vi "Rayleigh Inverse CDF.vi"(10 "b":dbl=3.0, 11 "cdf(x)":dbl=0.25) -> (0 "error":i32, 3 "x":dbl=2.275582849322796)   [LabVIEW 2010, in "NI_Gmath.lvlib"]
doc: "Computes the continuous inverse cumulative distribution function (CDF) of the various distributions. You must manually select the polymorphic instance to use."
uses:
  NI_Gmath.lvlib
  st_error_code.ctl
panel:
  # "Rayleigh Inverse CDF"
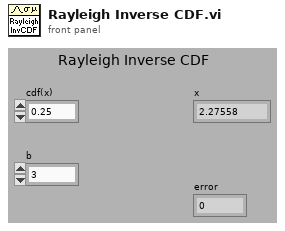
[diagram p1: front panel]
types:
  T1 = typedef "NI_Gmath.lvlib/st_error_code.ctl" = i32
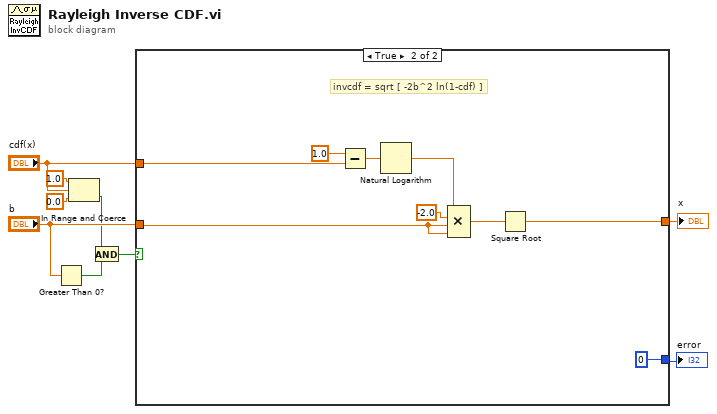
[diagram p0: block diagram]
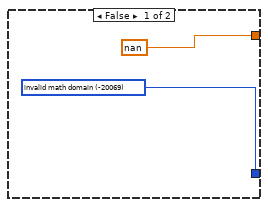
[diagram p2: hidden frame]
diagram:
  n1 = Greater Than 0?(x="b") -> (x > 0?=w3:bool)
  n2 = In Range and Coerce(upper limit=1.0, x="cdf(x)", lower limit=0.0) -> (In Range?=w2:bool)  [unwired: 1 out]
  n3 = And(x=w2, y=w3) -> (x .and. y?=w1:bool)
  n4 = case shown="True" w1 {
    tunnel: [w10 0 ("invalid math domain")] -> w9
    tunnel: [nan w19] -> w8
    tunnel: "cdf(x)" -> [_ w17]
    tunnel: "b" -> [_ w18]
    frame False {
      w10 = T1 -20069 items=["invalid math domain"=-20069, "Fourier interpolation size m >= n"=-20070, "empty array"=-20003] ("stat interp error code")
    }
    frame True {
      # "invcdf = sqrt [ -2b^2 ln(1-cdf) ]"
      n5 = Subtract(x=1.0, y=w17) -> (x-y=w14:dbl)
      n6 = Natural Logarithm(1:w14) -> (0:w13:dbl)
      n7 = Compound Arithmetic op=MULTIPLY(w13, -2.0 ("value"), w18, w18) -> (w12:dbl)
      n8 = Square Root(x=w12) -> (sqrt(x)=w19:dbl)
    }
  }
  "x" <- w8
  "error" <- w9
